vi "PENGUKURAN TINGGI BADAN.vi"() -> ()   [LabVIEW 2017]
uses:
  <vilib>/Instr/_visa.llb/VISA Configure Serial Port (Instr).vi
panel:
  out "HASIL REKAM TB":string
  out "NAMA PESERTA":string
  out "WAKTU REKAM":string
  out "TANGGAL REKAM":string
  in  "REKAM":bool
  in  "NAMA":string
  in  "stop":bool
  out "SERIAL MONITOR":string
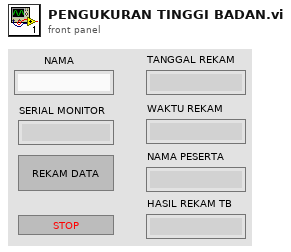
[diagram p1: front panel]
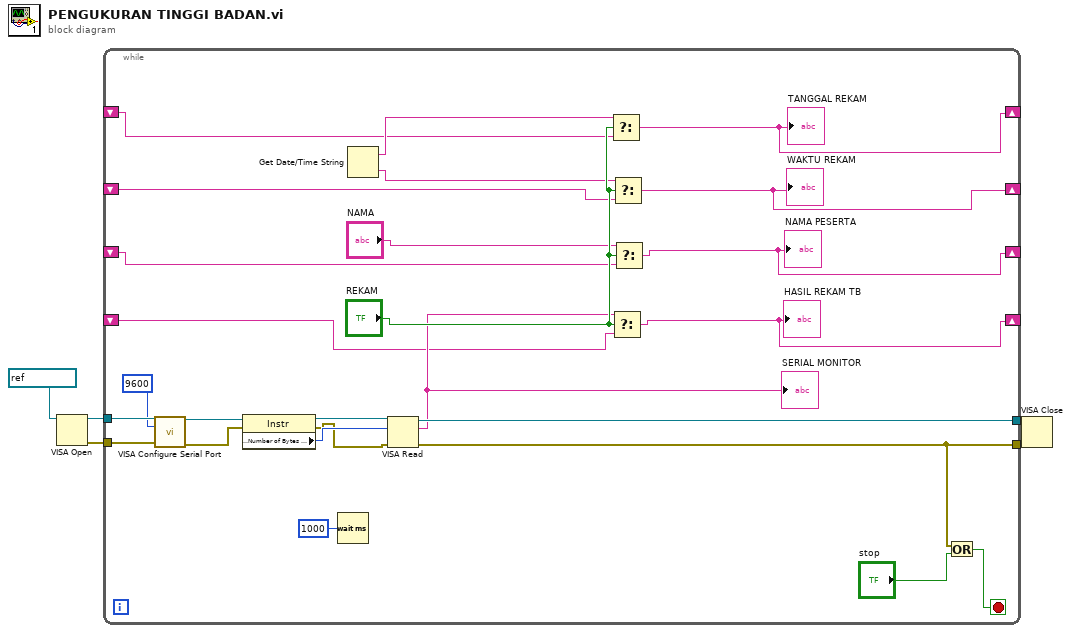
[diagram p0: block diagram]
diagram:
  n1 = VISA Open(VISA resource name=refnum<visa-resource-name> "COM15") -> (VISA resource name=w4:refnum<visa-resource-name>, error out=w3:errorcluster)  [unwired: 4 in]
  n2 = while {
    tunnel: w4 -> [w31]
    tunnel: w3 -> [w30]
    tunnel: [w23] -> w2
    tunnel: [w6] -> w1
    shift-right: [w17] -> _
    shift-left: _ -> [w9]
    shift-right: [w15] -> _
    shift-left: _ -> [w10]
    shift-right: [w19] -> _
    shift-left: _ -> [w11]
    shift-right: [w13] -> _
    shift-left: _ -> [w12]
    stop <- w8 stop-if-true
    n3 = call-poly "VISA Configure Serial Port"("VISA resource name"=w31, "baud rate (9600)"=u32 9600, "error in (no error)"=w30) -> ("VISA resource name out"=w28:refnum<visa-resource-name>, "error out"=w27:errorcluster)  [unwired: 11 in]
    n4 = property class="Instr"(reference=w28, error in=w27) -> (reference out=w26:refnum<visa-resource-name>, error out=w24:errorcluster, "Serial Settings:Number of Bytes at Serial Port"=w25:u32)
    n5 = Wait (ms)(milliseconds to wait=u32 1000) -> ()  [unwired: 1 out]
    n6 = Get Date/Time String() -> (date string=w18:string, time string=w16:string)  [unwired: 3 in]
    n7 = VISA Read(VISA resource name=w26, byte count=w25, error in (no error)=w24) -> (VISA resource name out=w23:refnum<visa-resource-name>, read buffer=w14:string, error out=w6:errorcluster)  [unwired: 1 out]
    "SERIAL MONITOR" <- w14
    n8 = Select(t=w18, s="REKAM", f=w9) -> (s? t:f=w17:string)
    "TANGGAL REKAM" <- w17
    n9 = Select(t=w14, s="REKAM", f=w12) -> (s? t:f=w13:string)
    "HASIL REKAM TB" <- w13
    n10 = Select(t=w16, s="REKAM", f=w10) -> (s? t:f=w15:string)
    "WAKTU REKAM" <- w15
    n11 = Select(t="NAMA", s="REKAM", f=w11) -> (s? t:f=w19:string)
    "NAMA PESERTA" <- w19
    n12 = Or(x=w6, y="stop") -> (x .or. y?=w8:bool)
  }
  n13 = VISA Close(VISA resource name=w2, error in (no error)=w1) -> ()  [unwired: 1 out]
